vi "Cluster Array Variant to Cluster Variant Array.vi"(0 "Variant":variant, 11 "error in (no error)":errorcluster) -> (4 "Array":variant[](array[variant]), 15 "error out":errorcluster)   [LabVIEW 2020]
uses:
  <vilib>/Utility/Data Type/NI_Data Type.lvlib
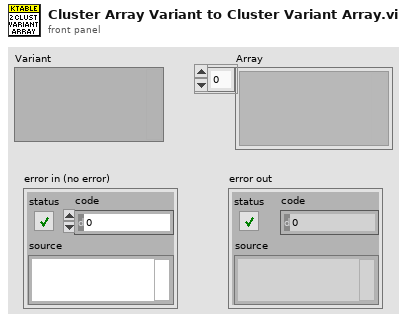
[diagram p1: front panel]
types:
  T1 = typedef "NI_Data Type.lvlib/Data Type.ctl" = enum8{"Invalid Type", "Void", "I8", "I16", "I32", "I64", "U8", "U16", "U32", "U64", "Single Float", "Double Float", "Extended Float", "Single Complex", "Double Complex", "Extended Complex", "Enum U8", "Enum U16", "Enum U32", "Enum U64", "Single Float With Unit", "Double Float With Unit", "Extended Float With Unit", "Single Complex with Unit", "Double Complex with Unit", "Extended Complex with Unit", "Boolean", "String", "Path", "Picture", "Tag", "Array", "Cluster", "Variant", "LV Variant", "Waveform", "Timestamp", "Digital Waveform", "Digital Data", "ExpressData", "Refnum", "External Data", "VI", "Poly VI", "LabVIEW Class Instance", "Fixed Point", "Set Collection", "Map Collection"}
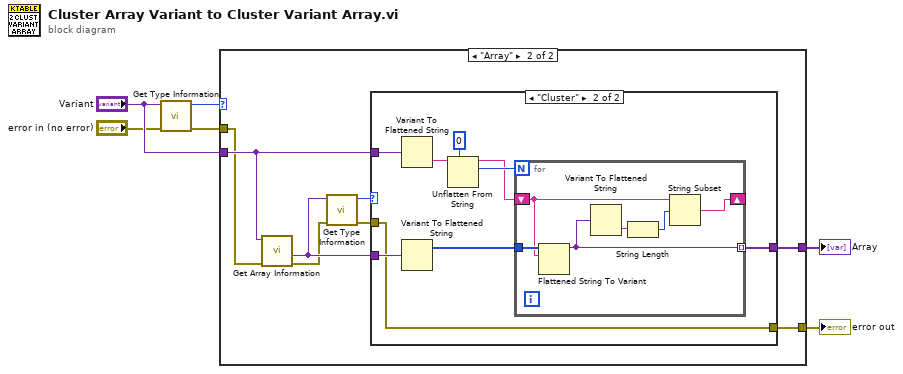
[diagram p0: block diagram]
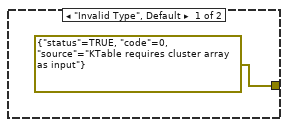
[diagram p2: hidden frame]
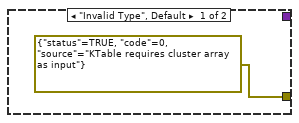
[diagram p3: hidden frame]
diagram:
  n1 = call <vilib>:"Get Type Information.vi"("error in (no error)"="error in (no error)", "variant"="Variant") -> ("error out"=w2:errorcluster, "type"=w4:T1)  [unwired: 5 in, 3 out]
  n2 = case shown="\"Array\"" w4 {
    tunnel: [_ w15] -> w6
    tunnel: "Variant" -> [_ w13]
    tunnel: w2 -> [_ w12]
    tunnel: [errorcluster {"status"=TRUE, "code"=0, "source"="KTable requires cluster array as input"} ("error out") w8] -> w1
    frame "Invalid Type", Default {
    }
    frame "Array" {
      n3 = call <vilib>:"Get Array Information.vi"("error in (no error)"=w12, "variant"=w13) -> ("error out"=w11:errorcluster, "array element data type"=w14:variant)  [unwired: 6 in, 2 out]
      n4 = call <vilib>:"Get Type Information.vi"("error in (no error)"=w11, "variant"=w14) -> ("error out"=w9:errorcluster, "type"=w10:T1)  [unwired: 5 in, 3 out]
      n5 = case shown="\"Cluster\"" w10 {
        tunnel: [_ w25] -> w15
        tunnel: w14 -> [_ w22]
        tunnel: w13 -> [_ w21]
        tunnel: w9 -> [_ w17]
        tunnel: [errorcluster {"status"=TRUE, "code"=0, "source"="KTable requires cluster array as input"} ("error out") w17] -> w8
        frame "Invalid Type", Default {
        }
        frame "Cluster" {
          n6 = Variant To Flattened String(Variant=w21) -> (data string=w18:string)  [unwired: 1 out]
          n7 = Variant To Flattened String(Variant=w22) -> (1:w23:i16[])  [unwired: 1 out]
          n8 = Unflatten From String(type=0, binary string=w18) -> (rest of the binary string=w20:string, value=w24:i32)  [unwired: 3 in, 1 out]
          n9 = for {
            N: w24 -> [_]
            tunnel: w23 -> [w31]
            shift-right: [w28] -> _
            shift-left: w20 -> [w26]
            tunnel: [w27] -> w25 mode=indexing
            n10 = Flattened String To Variant(6:w26, 7:w31) -> (3:w27:variant)  [unwired: 1 in, 1 out]
            n11 = Variant To Flattened String(Variant=w27) -> (data string=w29:string)  [unwired: 1 out]
            n12 = String Length(string=w29) -> (length=w30:i32)
            n13 = String Subset(string=w26, offset (0)=w30) -> (substring=w28:string)  [unwired: 1 in]
          }
        }
      }
    }
  }
  "Array" <- w6
  "error out" <- w1
